vi "PhotonPoseEstimator_CalcDifference.vi"(9 "Y_Pose3":T1={"Translation3d"={"X"=0.0, "Y"=0.0, "Z"=0.0}, "Rotation3d"={"Q_quaternion"={"R"=1.0, "V"=[0.0, 0.0, 0.0]}}} {"Translation3d"."Z" format="%14.3f"; "Translation3d"."Y" format="%14.3f"; "Translation3d"."X" format="%14.3f"}, 11 "X_Pose3":T1={"Translation3d"={"X"=0.0, "Y"=0.0, "Z"=0.0}, "Rotation3d"={"Q_quaternion"={"R"=1.0, "V"=[0.0, 0.0, 0.0]}}} {"Translation3d"."Z" format="%14.3f"; "Translation3d"."Y" format="%14.3f"; "Translation3d"."X" format="%14.3f"}) -> (3 "Difference":dbl)   [LabVIEW 2019, in "PhotonVisionLib.lvlib"]
doc: "This is an internal function. Use Update or Update_Pipeline instead of this function.\n\nIt calculates an overall difference between two poses. Difference is defined as the vector magnitude between the two poses"
uses:
  PhotonVisionLib.lvlib
  <vilib>/Rock Robotics/WPI/ThirdParty/JAS_Junk/TrajLib/TypeDef/POSE3D.ctl
  <vilib>/Rock Robotics/WPI/ThirdParty/JAS_Junk/TrajLib/TypeDef/TRANSLATION3D.ctl
  <vilib>/Rock Robotics/WPI/ThirdParty/JAS_Junk/TrajLib/TypeDef/ROTATION3D.ctl
  <vilib>/Rock Robotics/WPI/ThirdParty/JAS_Junk/TrajLib/TypeDef/QUATERNION.ctl
  <vilib>/Rock Robotics/WPI/ThirdParty/JAS_Junk/TrajLib/Trajectory_Library.lvlib
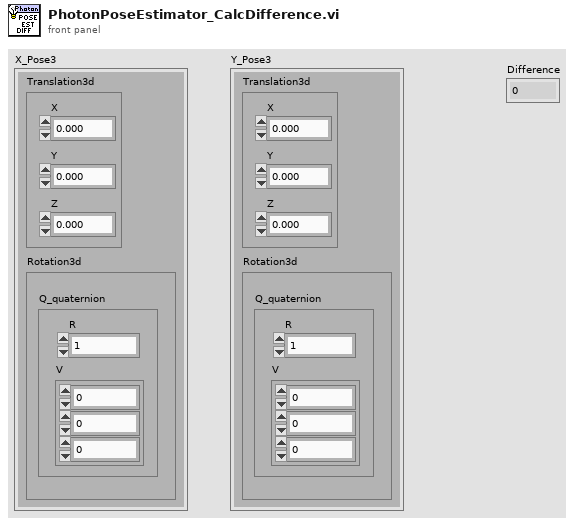
[diagram p1: front panel]
types:
  T1 = typedef "Trajectory_Library.lvlib/POSE3D.ctl" = cluster{"Translation3d":T2, "Rotation3d":T3}
  T2 = typedef "Trajectory_Library.lvlib/TRANSLATION3D.ctl" = cluster{"X":dbl, "Y":dbl, "Z":dbl}
  T3 = typedef "Trajectory_Library.lvlib/ROTATION3D.ctl" = cluster{"Q_quaternion":T4}
  T4 = typedef "Trajectory_Library.lvlib/QUATERNION.ctl" = cluster{"R":dbl, "V":dbl[]}
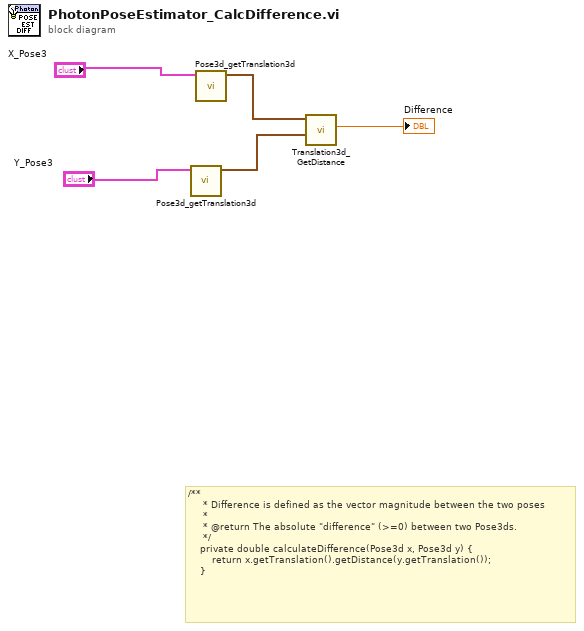
[diagram p0: block diagram]
diagram:
  # "/**\n     * Difference is defined as the vector magnitude between the two poses\n     *\n     * @return The absolute \"difference\" (>=0) between two Pose3ds.\n     */\n    private double calculateDifference(Pose3d x, Pose3d y) {\n        return x.getTranslation().getDistance(y.getTranslation());\n    }"
  n1 = call <vilib>:"Pose3d_getTranslation3d.vi"("in Pose3d"="Y_Pose3") -> ("out Translation3d"=w2:T2)  [unwired: 10 in]
  n2 = call <vilib>:"Pose3d_getTranslation3d.vi"("in Pose3d"="X_Pose3") -> ("out Translation3d"=w3:T2)  [unwired: 10 in]
  n3 = call <vilib>:"Translation3d_GetDistance.vi"("other Translation3d"=w2, "In Translation3d"=w3) -> ("Distance"=→"Difference":dbl)  [unwired: 9 in]
